vi "load binaries from file.vi"(8 "error in (no error)":errorcluster, 11 "manager_daemon in":refnum<class "manager_daemon.lvclass">) -> (0 "error out":errorcluster, 3 "manager_daemon out":refnum<class "manager_daemon.lvclass">)   [LabVIEW 2024, in "manager_daemon.lvclass"]
uses:
  manager_daemon.lvclass
  manager_daemon.lvclass/manager_daemon.ctl
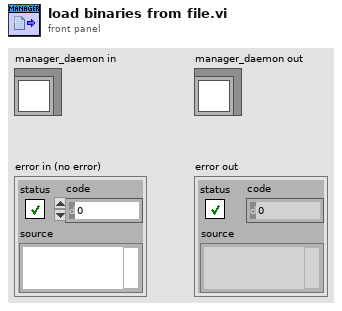
[diagram p1: front panel]
types:
  T1 = typedef "manager_daemon.lvclass/PublisherMap--map.ctl" = map{string, T2}
  T2 = typedef "manager_daemon.lvclass/PublisherData--cluster.ctl" = cluster{"id":i32, "volumes":set{i32}}
  T3 = typedef "manager_daemon.lvclass/IssueData--clustrer.ctl" = cluster{"cover_date":timestamp, "cv_id":string, "name":string, "sortable_name":string, "issue_number":string, "deck":string, "description":string, "volume id":i32, "store_date":timestamp, "date_last_updated":timestamp, "site_detail_url":string, "cover_url":string, "source_path":path, "in_collection":bool, "display_date":timestamp}
  T4 = typedef "manager_daemon.lvclass/sub-map--map.ctl" = map{string, T5}
  T5 = typedef "manager_daemon.lvclass/SubData--cluster.ctl" = cluster{"id":i32, "issues":set{i32}}
  T6 = typedef "manager_daemon.lvclass/VolumeData--cluster.ctl" = cluster{"name":string, "sortable_name":string, "aliases":string[], "description":string, "site_detail_url":string, "count_of_issues":i32, "start_year":i32, "publisher_id":i32, "issue_ids":i32[], "date_last_updated":timestamp, "volume":i32, "cv_id":string, "volume type":T7, "source_path":path}
  T7 = typedef "CV_Shared_Library.lvlib/volume.type--enum.ctl" = enum16{"Ongoing", "Limited Series", "Annual", "One Shot", "Reprint/Document", "Star Comics", "Epic Comics"}
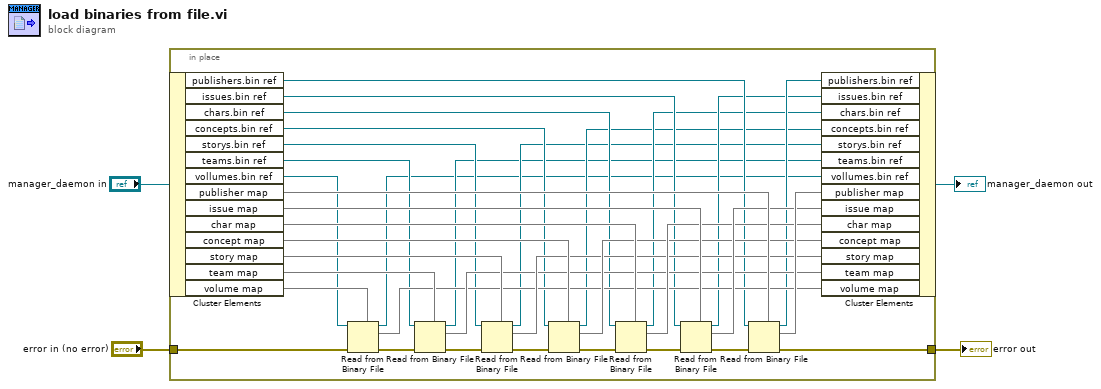
[diagram p0: block diagram]
diagram:
  n1 = in-place {
    in-place-border: "error in (no error)" -> [w19]
    in-place-border: [w12] -> w2
    n2 = in-place-cluster #1("manager_daemon in") -> ("publishers.bin ref"=w20:refnum<file>, "issues.bin ref"=w21:refnum<file>, "chars.bin ref"=w22:refnum<file>, "concepts.bin ref"=w23:refnum<file>, "storys.bin ref"=w24:refnum<file>, "teams.bin ref"=w25:refnum<file>, "vollumes.bin ref"=w26:refnum<file>, "publisher map"=w34:T1, "issue map"=w35:map{i32, T3}, "char map"=w36:T4, "concept map"=w37:T4, "story map"=w38:T4, "team map"=w39:T4, "volume map"=w40:map{i32, T6})
    n3 = Read from Binary File(5:w40, 8:w19, 11:w26) -> (0:w18:errorcluster, 2:w27:map{i32, T6}, 3:w5:refnum<file>)  [unwired: 3 in, 1 out]
    n4 = Read from Binary File(5:w39, 8:w18, 11:w25) -> (0:w17:errorcluster, 2:w28:T4, 3:w6:refnum<file>)  [unwired: 3 in, 1 out]
    n5 = Read from Binary File(5:w38, 8:w17, 11:w24) -> (0:w16:errorcluster, 2:w29:T4, 3:w7:refnum<file>)  [unwired: 3 in, 1 out]
    n6 = Read from Binary File(5:w37, 8:w16, 11:w23) -> (0:w15:errorcluster, 2:w30:T4, 3:w8:refnum<file>)  [unwired: 3 in, 1 out]
    n7 = Read from Binary File(5:w36, 8:w15, 11:w22) -> (0:w14:errorcluster, 2:w31:T4, 3:w9:refnum<file>)  [unwired: 3 in, 1 out]
    n8 = Read from Binary File(5:w35, 8:w14, 11:w21) -> (0:w13:errorcluster, 2:w32:map{i32, T3}, 3:w10:refnum<file>)  [unwired: 3 in, 1 out]
    n9 = Read from Binary File(5:w34, 8:w13, 11:w20) -> (0:w12:errorcluster, 2:w33:T1, 3:w11:refnum<file>)  [unwired: 3 in, 1 out]
    n10 = in-place-cluster #1("publishers.bin ref"=w11, "issues.bin ref"=w10, "chars.bin ref"=w9, "concepts.bin ref"=w8, "storys.bin ref"=w7, "teams.bin ref"=w6, "vollumes.bin ref"=w5, "publisher map"=w33, "issue map"=w32, "char map"=w31, "concept map"=w30, "story map"=w29, "team map"=w28, "volume map"=w27) -> (→"manager_daemon out":refnum<class "manager_daemon.lvclass">)
  }
  "error out" <- w2
